vi "Aurora Send TX trigger data.vi"(0 "start trigger":bool, 5 "aurora.write":bool, 7 "aurora.reset trigger":bool, 13 "clear overflow":bool, 14 "aurora tx fifo":refnum<k21>) -> (4 "tx overflow latch":bool, 6 "trig count":u16)   [LabVIEW 2019, in "FPGA Utility.lvlib"]
uses:
  FPGA Utility.lvlib
  <vilib>/rvi/Emulation/niFpgaSctlEmulationGetInTimedLoop.vi
  <vilib>/Utility/error.llb/Clear Errors.vi
  <instrlib>/_niInstr/Basic Elements/v1/FPGA/Private/Count Up U16.vi
  <vilib>/rvi/DataTransferAndStorage/Container/Common/niFpgaContainerExecOnDevCompGetState.vi
  <vilib>/rvi/Emulation/niFpgaEmulationIsFPGAContextNoSignature.vi
  <vilib>/rvi/errors/niFpgaSetErrorForExecOnDevCompSimple.vi
  <vilib>/rvi/eio/common/nirviEmuReportErrorAndStop.vi
  <vilib>/rvi/DataTransferAndStorage/Container/Common/niFpgaContainerGetUniqueNameForEmu.vi
  <vilib>/rvi/FIFO/Fifo_Resource/nirvififoEmulationSetSize.vi
  <vilib>/rvi/FIFO/Fifo_Resource/nirviFifoEmulationQueueMgr.vi
  <instcachedir>/0/nirviFifoEmulationQueueMgr_E5CAEC123FF24DC58D834DCA3CDAA9B5.lvgen/nirviFifoEmulationQueueMgr_E5CAEC123FF24DC58D834DCA3CDAA9B5_008.vi
  <vilib>/rvi/FIFO/Fifo_Resource/nirvififoEmulationDetermineInputValidOut.vi
  <vilib>/rvi/FIFO/Fifo_Resource/nirvififoEmulationCreateLock.vi
  <vilib>/rvi/Emulation/niFpgaProcessEmulError.vi
  <vilib>/rvi/FIFO/Fifo_Resource/nirvififoEmulationObtainLock.vi
  <vilib>/rvi/FIFO/Fifo_Resource/nirvififoEmulationReleaseLock.vi
  <vilib>/rvi/occurrence/nirviWaitOnOccurrenceBase.vi
  <vilib>/rvi/errors/nirviReportUnexpectedCaseInternalError.vi
  <vilib>/rvi/errors/nirviReportUnexpectedCaseInternalError (U32).vi
  <vilib>/rvi/interface/RandomDataEmulation/niFpgaRandomDataHandleErrors.vi
  <vilib>/rvi/DataTransferAndStorage/Container/XNode/niFpgaContainer.xnode
  <vilib>/rvi/FIFO/Fifo_Resource/niFpgaFifoEmulationRefIn.vi
  <instrlib>/_niInstr/Basic Elements/v1/FPGA/niInstr Basic Elements v1 FPGA.lvlib
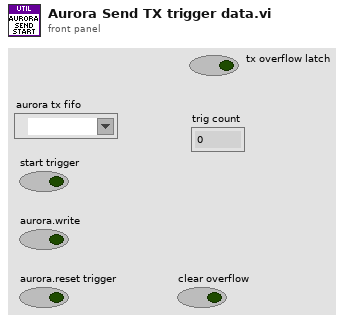
[diagram p1: front panel]
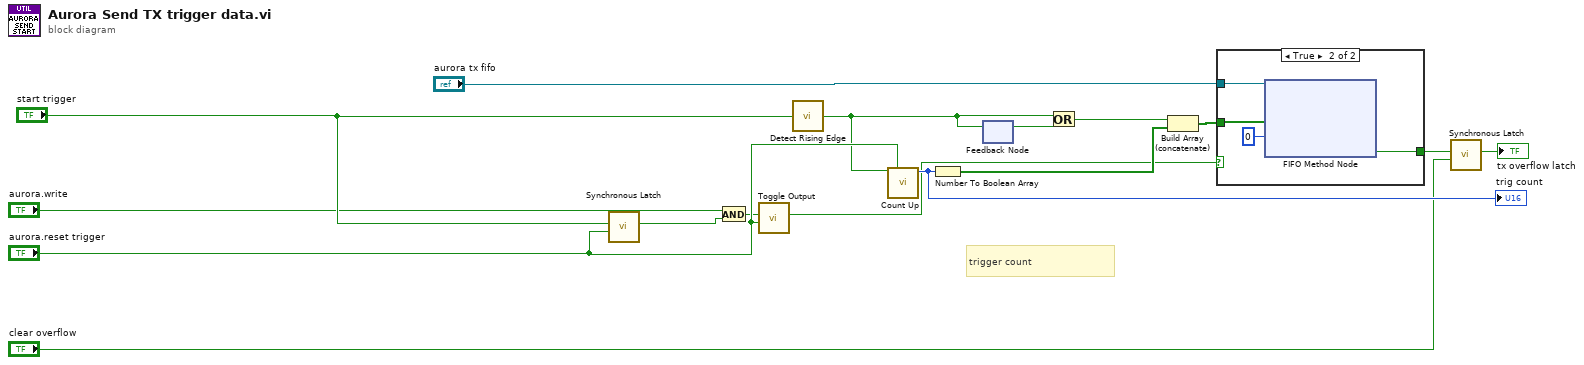
[diagram p0: block diagram]
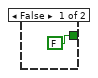
[diagram p2: hidden frame]
diagram:
  # "trigger count"
  n1 = call <instrlib>:"Synchronous Latch.vi"("clear"="aurora.reset trigger", "set"="start trigger") -> ("out"=w3:bool)  [unwired: 9 in]
  n2 = And(x="aurora.write", y=w3) -> (x .and. y?=w1:bool)
  n3 = call <instrlib>:"Toggle Output.vi"("clear"="aurora.reset trigger", "toggle"=w1) -> ("output"=w7:bool)  [unwired: 9 in]
  n4 = call <instrlib>:"Detect Rising Edge.vi"("signal"="start trigger") -> ("edge detected"=w11:bool)  [unwired: 14 in]
  n5 = call-poly <instrlib>:"Count Up.vi"("increment"=w11, "reset"="aurora.reset trigger") -> ("count out"=w12:u16)  [unwired: 13 in]
  "trig count" <- w12
  n6 = Number To Boolean Array(number=w12) -> (Boolean array=w15:bool[])
  n7 = feedback #1() -> (w8:bool)  [unwired: 1 in]
  n8 = feedback-in #1(w11) -> ()
  n9 = Or(x=w11, y=w8) -> (x .or. y?=w9:bool)
  n10 = Build Array (concatenate)(w9, w15) -> (w10:bool[])
  n11 = case shown="True" w7 {
    tunnel: [FALSE ("Timed Out?") w21] -> w5
    tunnel: w10 -> [_ w20]
    tunnel: "aurora tx fifo" -> [_ w18]
    frame False {
    }
    frame True {
      n12 = xnode ("FIFO Method Node")("Element"=w20, "Timeout"=0, "FIFO In"=w18) -> ("Timed Out?"=w21:bool)  [unwired: 1 out]
    }
  }
  n13 = call <instrlib>:"Synchronous Latch.vi"("clear"="clear overflow", "set"=w5) -> ("out"=→"tx overflow latch":bool)  [unwired: 9 in]
